vi "Get Sequence.vi"(8 "error in (no error)":errorcluster, 11 "Sequencer in":refnum<class "Sequencer.lvclass">) -> (0 "error out":errorcluster, 3 "Sequence":refnum<class "Sequence.lvclass">)   [LabVIEW 2024, in "Ramses Sequencer.lvlib" / "Sequencer.lvclass"]
uses:
  Sequencer.lvclass
  C:/Program Files (x86)/Enterative/Ramses Framework/Ramses Framework.lvlibp/Service/Service.lvclass
  Sequence/Sequence.lvclass
  Program Files (x86)/Enterative/Ramses Framework/Ramses Framework.lvlibp/Service/Service.lvclass
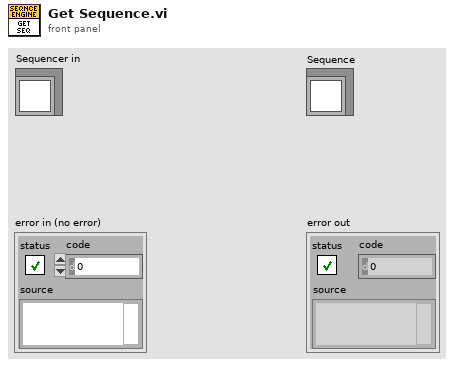
[diagram p1: front panel]
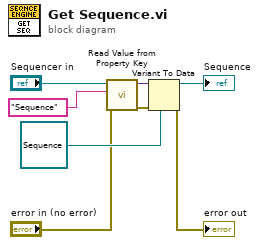
[diagram p0: block diagram]
diagram:
  n1 = call "Read Value from Property Key.vi"("error in (no error)"="error in (no error)", "Key"="Sequence", "Service in"="Sequencer in") -> ("error out"=w4:errorcluster, "Value"=w3:variant)  [unwired: 7 in]
  n2 = Variant To Data(error in=w4, type=refnum<class "Sequence.lvclass"> refnum ("Sequence"), Variant=w3) -> (data=→"Sequence":refnum<class "Sequence.lvclass">, error out=→"error out":errorcluster)
